vi "Leitura_de_Arquivo.vi"() -> ()   [LabVIEW 2012]
panel:
  out "text":string
  in  "OK Button":bool
  in  "file path (use dialog)":path
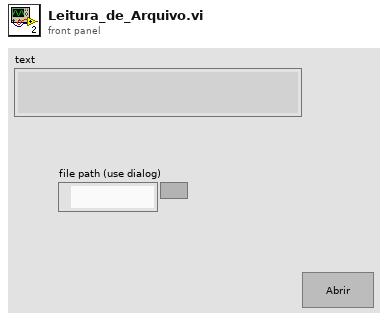
[diagram p1: front panel]
types:
  T1 = enum16{"open", "replace", "create", "open or create", "replace or create", "replace or create with confirmation"}
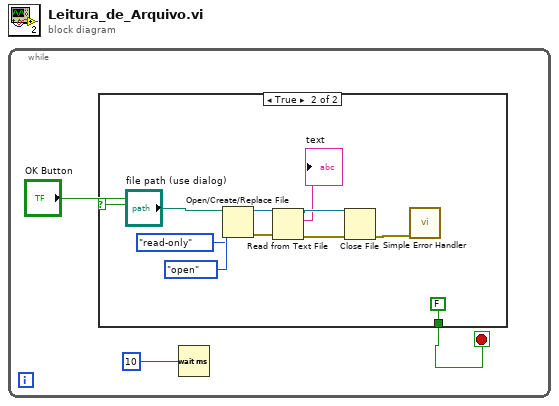
[diagram p0: block diagram]
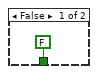
[diagram p2: hidden frame]
diagram:
  n1 = while {
    stop <- w1 stop-if-true
    n2 = case shown="True" "OK Button" {
      tunnel: [FALSE FALSE] -> w1
      frame False {
      }
      frame True {
        n3 = Open/Create/Replace File(file path (use dialog)="file path (use dialog)", operation (0:open)=T1."open", access (0:read/write)=enum16{"read/write", "read-only", "write-only"}."read-only") -> (refnum out=w6:refnum<file>, error out=w9:errorcluster)  [unwired: 3 in, 1 out]
        n4 = Read from Text File(file (use dialog)=w6, error in=w9) -> (refnum out=w7:refnum<file>, text=→"text":string, error out=w8:errorcluster)  [unwired: 2 in, 1 out]
        n5 = Close File(refnum=w7, error in=w8) -> (error out=w14:errorcluster)  [unwired: 1 out]
        n6 = call <vilib>:"Simple Error Handler.vi"("error in (no error)"=w14) -> ()  [unwired: 4 in, 5 out]
      }
    }
    n7 = Wait (ms)(milliseconds to wait=10) -> ()  [unwired: 1 out]
  }
